vi "Dashboard Main.vi"() -> ()   [LabVIEW 2017]
uses:
  <vilib>/Utility/miscctls.llb/LVRowAndColumnTypeDef.ctl
  <vilib>/event_ctls.llb/eventvkey.ctl
  <vilib>/Rock Robotics/Network Tables/NT Read Numeric Array.vi
  <vilib>/Rock Robotics/Network Tables/NT Read Boolean.vi
  <vilib>/Rock Robotics/WPI/Dashboard/WPI_DashboardLogging Global.vi
  <vilib>/vision/NI_Vision_Development_Module.lvlib
panel:
  in  "Camera Settings Right":T1={"Frame Rate"=30, "Compression"=30, "Size"=1, "DB Camera Config"=FALSE} {"Frame Rate" scale=1.0..30.0; "Compression" scale=100.0..-1.0; "Size" items=["640x480", "320x240", "160x120"]}
  in  "Camera Name Right":string(combo)="No Camera Selection"
  out "Camera Info":cluster{"Mbps LED":bool, "Mbps":dbl, "fps":dbl} {"fps" format="%#.1g"; "Mbps" format="%#.1g"}
  in  "Camera Settings":T1={"Frame Rate"=30, "Compression"=30, "Size"=1, "DB Camera Config"=FALSE} {"Frame Rate" scale=1.0..30.0; "Compression" scale=100.0..-1.0; "Size" items=["640x480", "320x240", "160x120"]}
  in  "TCP":refnum<k5>
  in  "Rec Mode":enum32{"Stop", "Record", "Playback"}(radio)
  out "Robot IP":string
  out "Image Message":string="Timeout in Camera Communications"
  in  "Dashboard Tab":T2(tab)
  in  "Select Auto":string(combo)="Select Autonomous ..."
  out "NT Connection":bool
  out "MotorChart R":cluster{"Numeric":dbl, "Numeric":dbl}(graph)
  out "MotorChart L":cluster{"Numeric":dbl, "Numeric":dbl}(graph)
  out "MotorSliders R":cluster{"MotorSlide1":dbl, "MotorSlide2":dbl} {"MotorSlide2" scale=-1.0..1.0 scale format="%#_2e"; "MotorSlide1" scale=-1.0..1.0 scale format="%#_2e"}
  out "MotorSliders L":cluster{"MotorSlide1":dbl, "MotorSlide2":dbl} {"MotorSlide2" scale=-1.0..1.0 scale format="%#_2e"; "MotorSlide1" scale=-1.0..1.0 scale format="%#_2e"}
  out "Gyro":dbl(knob) scale=0.0..360.0
  out "JS1 Z":dbl(slide) scale=-1.0..1.0 scale format="%#_2e"
  out "JS1 Graph":cluster{"X":dbl, "Y":dbl}[](graph)
  out "JS1 Buttons":T3
  out "JS2 Z":dbl(slide) scale=-1.0..1.0 scale format="%#_2e"
  out "JS2 Graph":cluster{"X":dbl, "Y":dbl}[](graph)
  out "JS2 Buttons":T3
  out "Mode":T4(ring)=enum."Auto Disabled"
  out "Camera Image Right":T5(plugin-control)
  in  "DB/String 9":string
  in  "DB/String 8":string
  in  "DB/String 7":string
  in  "DB/String 6":string
  in  "DB/String 5":string
  in  "DB/String 4":string
  in  "DB/String 3":string
  in  "DB/String 2":string
  in  "DB/String 1":string
  in  "DB/String 0":string
  in  "DB/Slider 0":dbl(slide) scale=0.0..5.0
  in  "DB/Slider 1":dbl(slide) scale=0.0..5.0
  in  "DB/Slider 2":dbl(slide) scale=0.0..5.0
  in  "DB/Slider 3":dbl(slide) scale=0.0..5.0
  out "DB/LED 3":bool
  out "DB/LED 2":bool
  out "DB/LED 1":bool
  out "DB/LED 0":bool
  in  "DB/Button 3":bool
  in  "DB/Button 2":bool
  in  "DB/Button 1":bool
  in  "DB/Button 0":bool caption="New Name"
  in  "Drive X-Axis Correction":dbl=-0.2
  out "UseLeftEncoder":bool
  out "RDrive Encoder":dbl
  out "Flip Active":bool
  in  "BackCamera Rotate":sgl min=-360 max=360 step=1 format="%#_3g"
  in  "FrontCamera Rotate":sgl min=-360 max=360 step=1 format="%#_3g"
  out "Arm Sensor":bool
  out "Belly Sensor":bool
  out "Arm Encoder":dbl
  out "Arm Switch":bool
  out "LDrive Encoder":dbl
  in  "Test Slider":dbl(slide) scale=0.0..100.0 scale format="%#_3g"
  in  "On/Off":bool caption="Solenoid"
  in  "Test Name":u16(ring) items=["Select the test to run..."]
  in  "Test Tree":string(tree)
  in  "Motor":cluster{"Value":dbl, "Enable":bool} {"Value" scale=-1.0..1.0 scale format="%#_3g"}
  out "Progress":T6 {"Test Progress" scale=0.0..100.0}
  in  "Rev/Fwd":cluster{"Forward":bool, "Reverse":bool}
  in  "Test Ring":u16(ring) items=["Monochrome", "Color"]
  out "Cmd Status":string
  in  "Execute Command":bool
  in  "Command Params":string[][](table)
  in  "Command Selection":i32(listbox)
  in  "CheckList":i32(listbox)
  out "Tree":string(tree)
  out "Camera Image":T5(plugin-control)
  out "Background":bool
  in  "Camera Name":string(combo)="No Camera Selection"
  # "HW"
  # "HW"
  # "Joysticks"
  # "Drive Motors"
  # "Front"
  # "Right"
  # "Left"
  # "Back"
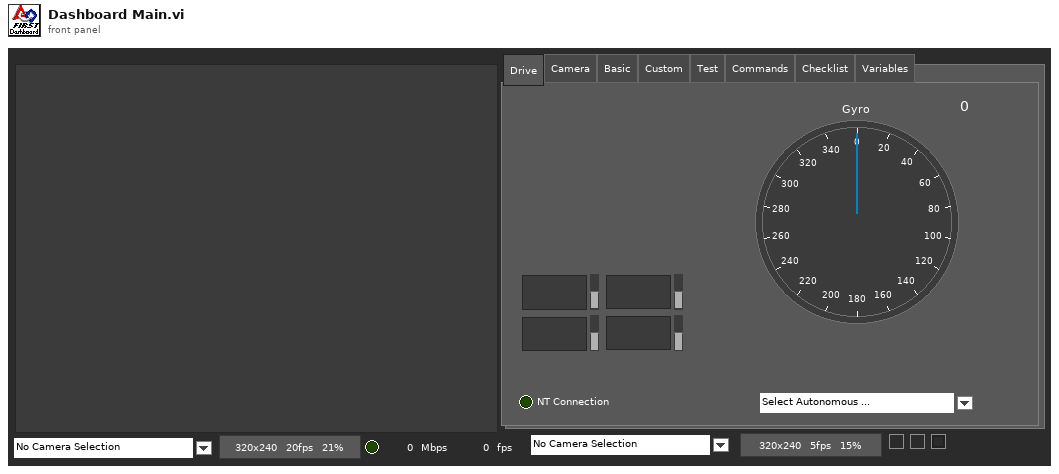
[diagram p1: front panel]
types:
  T1 = cluster{"Frame Rate":i32, "Compression":i32, "Size":u16, "DB Camera Config":bool}
  T2 = enum32{"Drive", "Camera", "Basic", "Custom", "Test", "Commands", "Checklist", "Variables"}
  T3 = cluster{bool, bool, bool, bool, bool, bool, bool, bool, bool, bool, bool, bool}
  T4 = enum8{"Tele-Op Disabled", "Tele-Op Enabled", "Auto Disabled", "Auto Enabled", "Test Disabled", "Test Enabled", "Disconnected", "No Code", "E-Stop"}
  T5 = typedef "IMAQ Image.ctl" = refnum<image>
  T6 = cluster{"Test Progress":u8, "Test Progress Text":string}
  T7 = cluster{"Save Path":path, "Interval (s)":dbl, "Keep":i32}
  T8 = typedef "Image Type" = u32
  T9 = cluster{"IDs":cluster{"RPC field ID":u16, "Unique ID":u16}, "String":string}
  T10 = cluster{string, string, "Saved DB Images Info":cluster{"Save Path":path, "Interval (s)":dbl, "Keep":i32}}
  T11 = cluster{"Camera Image":refnum<vi>, "Dashboard Tab":refnum<vi>, "Background":refnum<vi>, "Rec Mode":refnum<vi>, "Test Slider":refnum<vi>, "On/Off ":refnum<vi>, "Test Ring":refnum<vi>, "Rev/Fwd":refnum<vi>, "Test Name":refnum<vi>, "Motor":refnum<vi>, "Progress":refnum<vi>, "CheckList":refnum<vi>, "Tree":refnum<vi>, "Test Tree":refnum<vi>, "Command Params":refnum<vi>, "Command Selection":refnum<vi>, "Execute Command":refnum<vi>, "Cmd Status":refnum<vi>, "Camera Settings":refnum<vi>, "Camera Name":refnum<vi>, "Camera Info":refnum<vi>, "Camera Settings Right":refnum<vi>, "Camera Name Right":refnum<vi>, "Camera Image Right":refnum<vi>}
  T12 = cluster{"Error Strings":string, "Disable Counts":cluster{u16, u16}, "Rail Faults":cluster{u16, u16, u16}, "Robot IP":string, "DB Mode":u8, "Event Info":cluster{"Name":string, "Type":u8, "Number":u16, "Replay":u8}}
  T13 = cluster{"Storage":cluster{"Disk Free":u64, "RAM Block":u32, "RAM free":u32}, "CPU Utilization":cluster{"CPU % ISR":sgl, "CPU % Time Crit":sgl, "CPU % Timed Str":sgl, "CPU % High":sgl, "CPU % Above":sgl, "CPU % Normal":sgl, "CPU % Low":sgl}, "CAN":cluster{"% Bus Utilization":sgl, "Bus Off Cnt":u32, "TX_FIFO Full Cnt":u32, "Receive Error Cnt":u8, "Transmit Error Cnt":u8}, "HID":cluster{"HID Outputs":u32, "Rumble Low":u16, "Rumble High":u16}[]}
  T14 = cluster{"Status bits":cluster{"Test Mode":bool, "Autonomous":bool, "Enabled":bool, "Code Start":bool, "Brownout":bool, "Reserved 2":bool, "Reserved 3":bool, "E-Stop":bool}, "Code Trace":cluster{"Disabled":bool, "TeleOp":bool, "Auto":bool, "Test":bool}, "Controller Type":enum16{"unknown", "cRIO", "roboRio"}, "Code?":enum16{"unknown", "noCode", "code"}, "Battery V":dbl}
  T15 = cluster{"Control Bits":cluster{"TestMode":bool, "Autonomous":bool, "Enabled":bool, "FMS Present":bool, bool, bool, bool, "E-Stop":bool}, "Team Station ":u8, "Countdown":sgl, "Joystick Values":cluster{"Axes":dbl[], "Buttons":bool[], "POVs":i16[]}[]}
  T16 = cluster{"Axes":dbl[], "Buttons":bool[], "POVs":i16[]}[]
  T17 = cluster{"Axes":dbl[], "Buttons":bool[], "POVs":i16[]}
  T18 = cluster{"Buttons[0]":bool, "Buttons[1]":bool, "Buttons[2]":bool, "Buttons[3]":bool, "Buttons[4]":bool, "Buttons[5]":bool, "Buttons[6]":bool, "Buttons[7]":bool, "Buttons[8]":bool, "Buttons[9]":bool, "Buttons[10]":bool, "Buttons[11]":bool}
  T19 = cluster{"Camera Name Right":string, string, "Saved DB Images Info":cluster{"Save Path":path, "Interval (s)":dbl, "Keep":i32}}
  T20 = cluster{"Operation":enum16{"Update", "Clear"}, "Color Box":u32}[]
  T21 = typedef "eventvkey.ctl" = enum16{"ASCII", "Enter", "Return", "Shift", "Ctrl", "Alt", "Cmd", "Opt", "Caps", "NumLock", "Clear", "Break", "Up", "Down", "Left", "Right", "Insert", "Delete", "Home", "End", "PageUp", "PageDown", "Escape", "Help", "Pause", "ScrollLock", "F1", "F2", "F3", "F4", "F5", "F6", "F7", "F8", "F9", "F10", "F11", "F12", "F13", "F14", "F15", "F16", "F17", "F18", "F19", "F20", "F21", "F22", "F23", "F24", "Play", "VolumeUp", "VolumeDown", "Mute", "Two Byte Char"}
  T22 = cluster{"Image Size":bool, "Image Type":bool, "Pixel Value":bool, "ROI Information":bool, "Zoom Factor":bool}
  T23 = cluster{"Operation":enum16{"Update", "Clear"}, "Color Box":u32}
  T24 = typedef "LVRowAndColumnTypeDef.ctl" = cluster{"Row":i32, "Column":i32}
  T25 = cluster{"Shift":bool, "Ctrl":bool, "Alt":bool, "Cmd":bool, "Opt":bool}
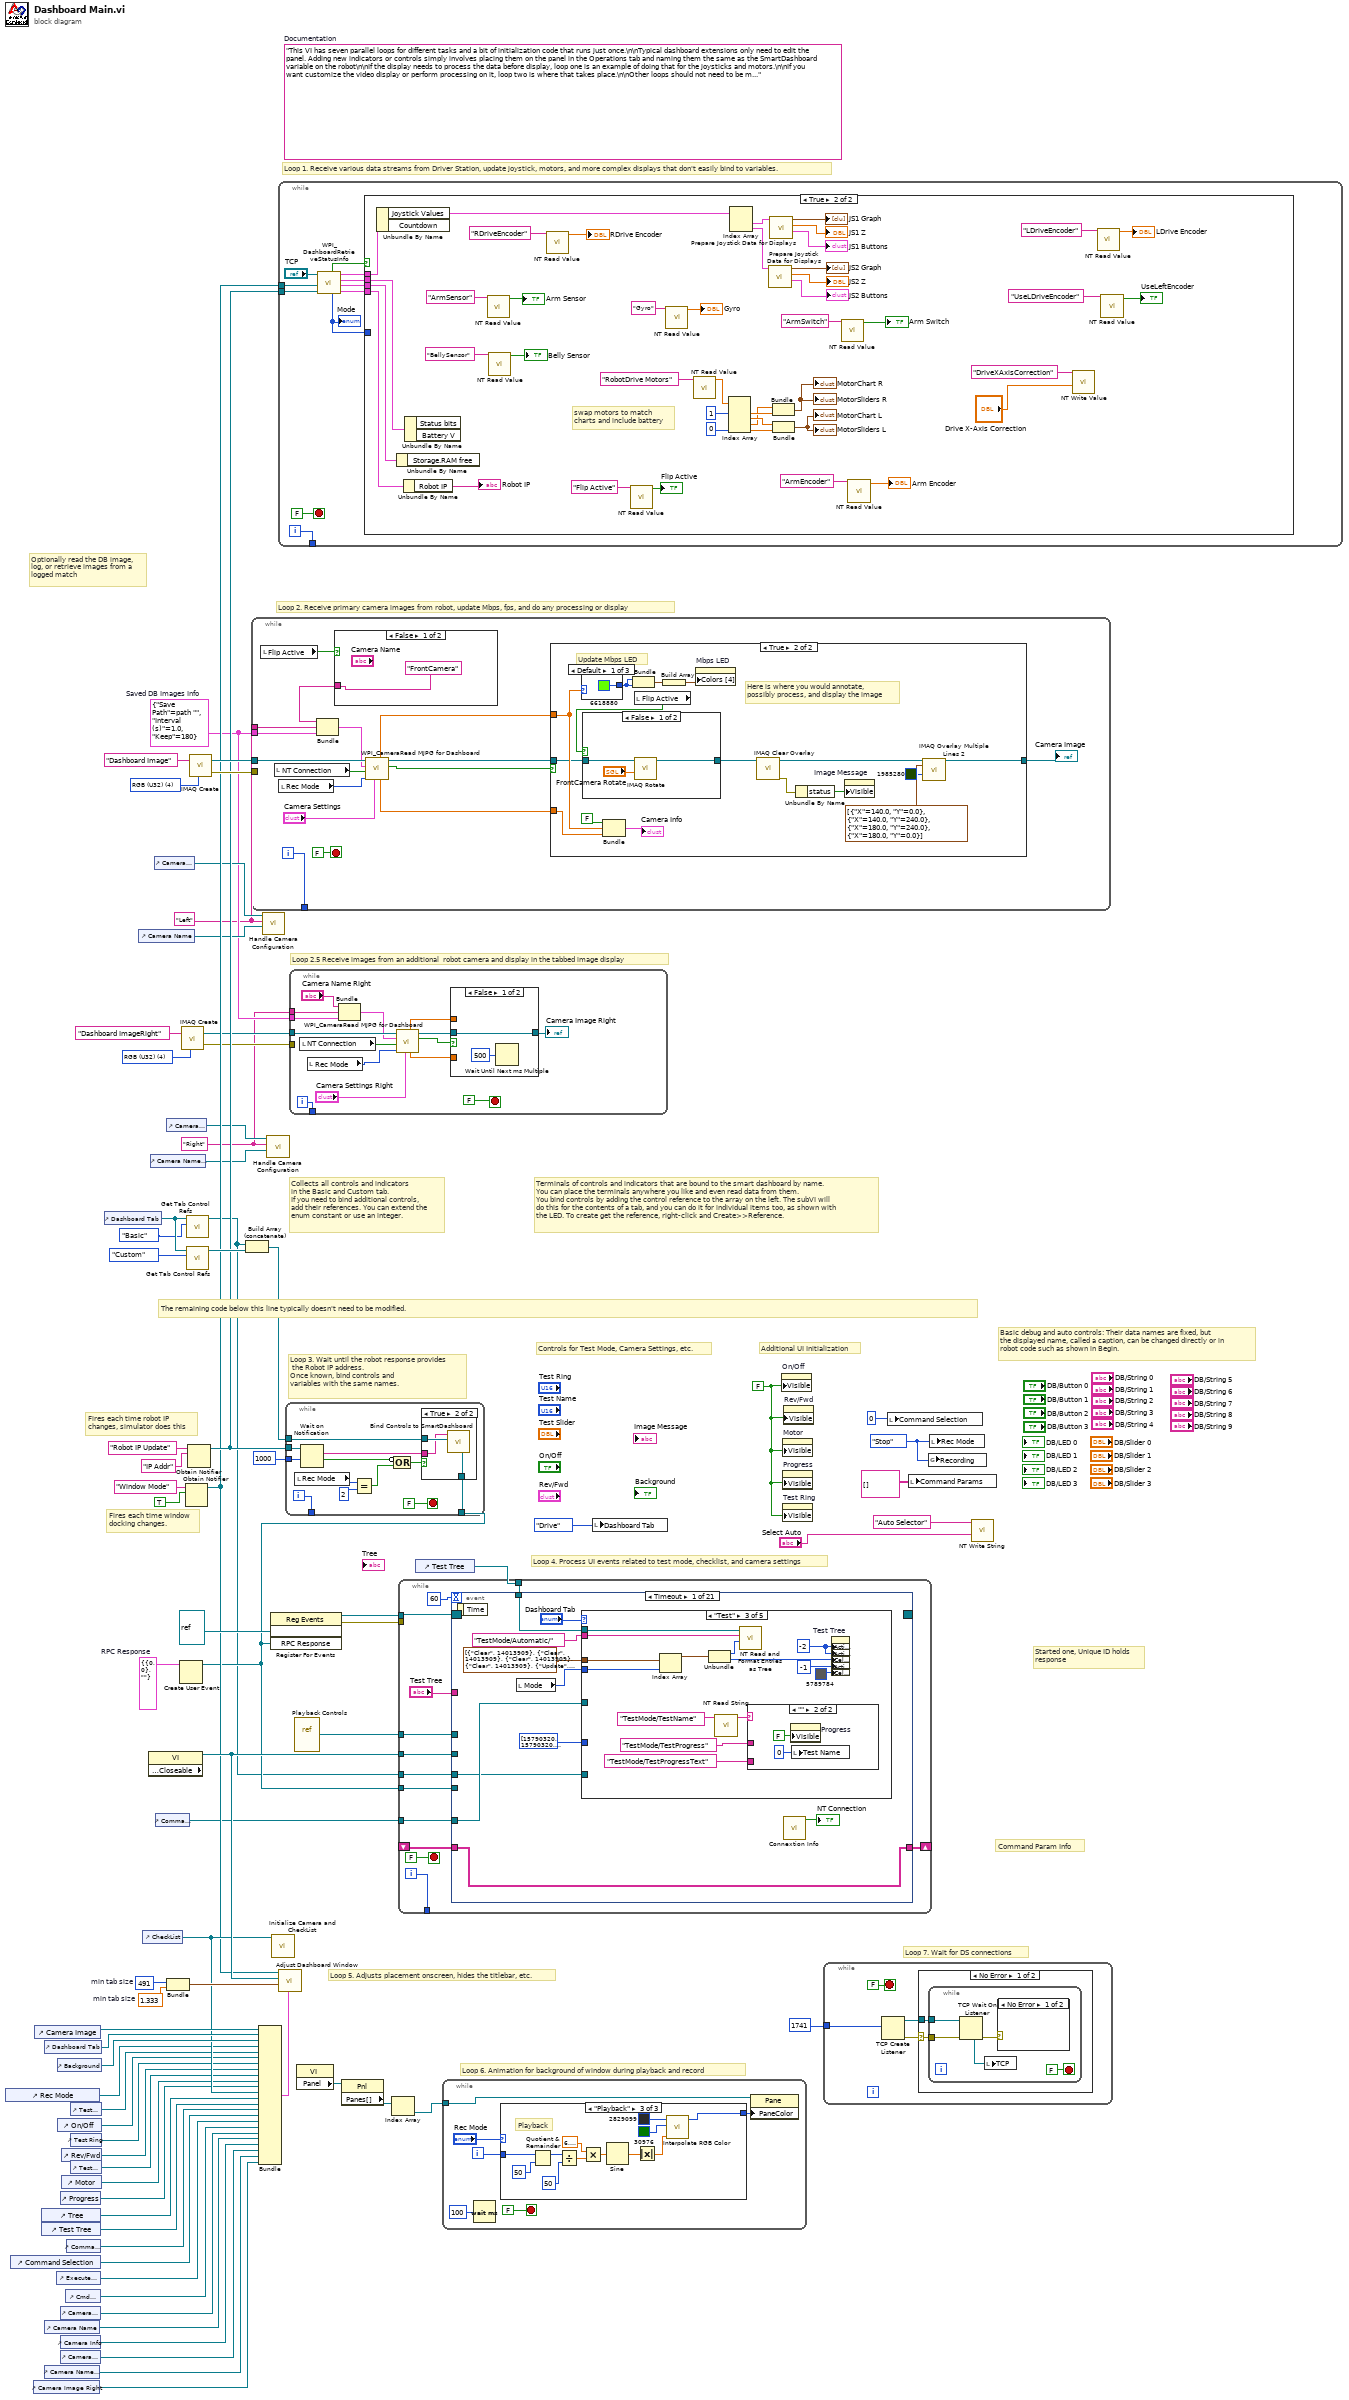
[diagram p0: block diagram]
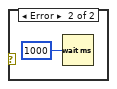
[diagram p3: hidden frame]
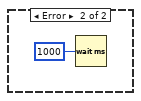
[diagram p4: hidden frame]
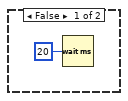
[diagram p5: hidden frame]
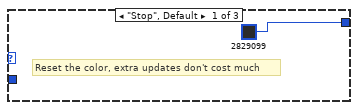
[diagram p6: hidden frame]
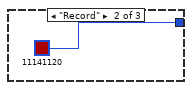
[diagram p7: hidden frame]
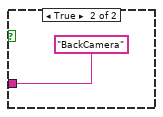
[diagram p9: hidden frame]
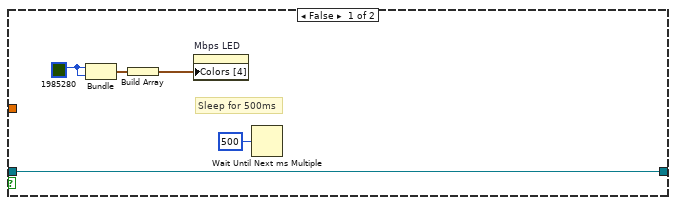
[diagram p10: hidden frame]
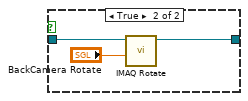
[diagram p11: hidden frame]
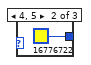
[diagram p12: hidden frame]
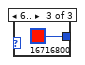
[diagram p13: hidden frame]
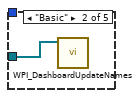
[diagram p15: hidden frame]
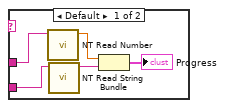
[diagram p16: hidden frame]
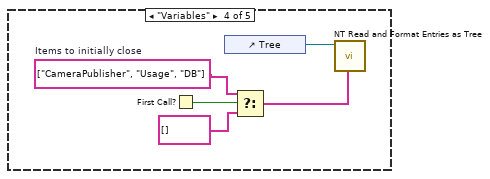
[diagram p17: hidden frame]
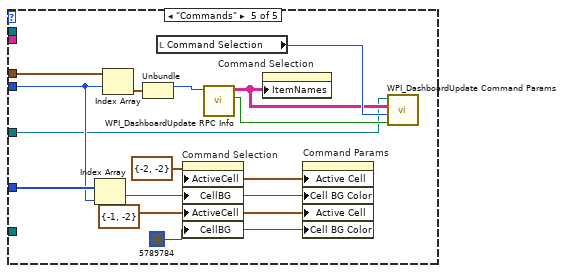
[diagram p18: hidden frame]
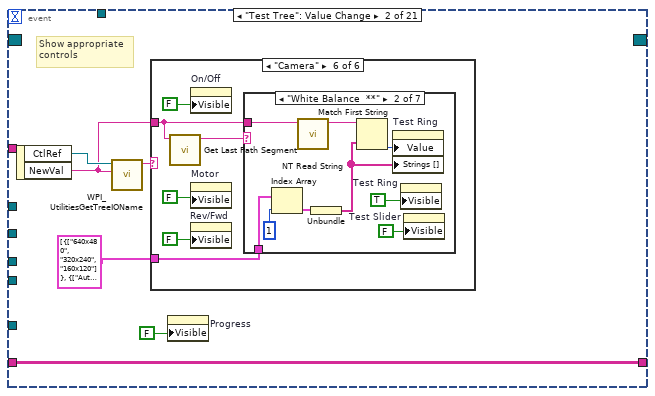
[diagram p19: hidden frame]
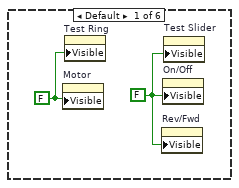
[diagram p20: hidden frame]
diagram:
  w4 = T7 {"Save Path"=path "", "Interval (s)"=1.0, "Keep"=180}  # Saved DB Images Info
  w3 = "Right"
  w2 = "Left"
  w14 = T8 4 items=["Grayscale (U8)", "Grayscale (I16)", "Grayscale (SGL)", "Complex (CSG)", "RGB (U32)", "HSL (U32)", "RGB (U64)"] ("Image Type")
  w29 = T9 {"IDs"={"RPC field ID"=0, "Unique ID"=0}, "String"=""}  # RPC Response
  w52 = 491  # min tab size
  w51 = 1.333  # min tab size
  w59 = enum32{"Stop", "Record", "Playback"}."Stop" ("Rec Mode")
  w36 = FALSE ("Visible")
  (unwired) "This VI has seven parallel loops for different tasks and a bit of initialization code that runs just once.\n\nTypical dashboard extensions only need to edit the panel. Adding new indicators or controls simply involves placing them on the panel in the Operations tab and naming them the same as the SmartDashboard variable on the robot\n\nIf the display needs to process the data before display, loop one is an example of doing that for the joysticks and motors.\n\nIf you want customize the video display or perform processing on it, loop two is where that takes place.\n\nOther loops should not need to be modified. They are pretty standard, and document the task they perform."  # Documentation
  w76 = T8 4 items=["Grayscale (U8)", "Grayscale (I16)", "Grayscale (SGL)", "Complex (CSG)", "RGB (U32)", "HSL (U32)", "RGB (U64)"] ("Image Type")
  # "Optionally read the DB image,\nlog, or retrieve images from a\nlogged match"
  # "Loop 2.5 Receive images from an additional  robot camera and display in the tabbed image display"
  # "Command Param Info"
  # "Started one, Unique ID holds\nresponse"
  # "Loop 7. Wait for DS connections"
  # "Basic debug and auto controls: Their data names are fixed, but\nthe displayed name, called a caption, can be changed directly or in\nrobot code such as shown in Begin."
  # "Controls for Test Mode, Camera Settings, etc."
  # "Additional UI Initialization"
  # "Loop 6. Animation for background of window during playback and record"
  # "Fires each time robot IP\nchanges, simulator does this"
  # "Fires each time window\ndocking changes."
  # "Collects all controls and indicators\nin the Basic and Custom tab.\nIf you need to bind additional controls,\nadd their references. You can extend the\nenum constant or use an integer."
  # "The remaining code below this line typically doesn't need to be modified."
  # "Loop 4. Process UI events related to test mode, checklist, and camera settings"
  # "Terminals of controls and indicators that are bound to the smart dashboard by name.\nYou can place the terminals anywhere you like and even read data from them.\nYou bind controls by adding the control reference to the array on the left. The subVI will\ndo this for the contents of a tab, and you can do it for individual items too, as shown with\nthe LED. To create get the reference, right-click and Create>>Reference."
  # "Loop 3. Wait until the robot response provides\n the Robot IP address.\nOnce known, bind controls and\nvariables with the same names."
  # "Loop 5. Adjusts placement onscreen, hides the titlebar, etc."
  # "Loop 1. Receive various data streams from Driver Station, update joystick, motors, and more complex displays that don't easily bind to variables."
  # "Loop 2. Receive primary camera images from robot, update Mbps, fps, and do any processing or display"
  n1 = control-ref of="Rec Mode"() -> (w42:refnum<vi>)
  n2 = control-ref of="Command Selection"() -> (w28:refnum<vi>)
  n3 = control-ref of="Camera Image Right"() -> (w7:refnum<vi>)
  n4 = control-ref of="Camera Image"() -> (w54:refnum<vi>)
  n5 = control-ref of="Tree"() -> (w46:refnum<vi>)
  n6 = control-ref of="Test Tree"() -> (w45:refnum<vi>)
  n7 = control-ref of="Dashboard Tab"() -> (w53:refnum<vi>)
  n8 = control-ref of="Camera Name"() -> (w19:refnum<vi>)
  n9 = control-ref of="Camera Name Right"() -> (w8:refnum<vi>)
  n10 = control-ref of="Execute Command"() -> (w30:refnum<vi>)
  n11 = control-ref of="Background"() -> (w49:refnum<vi>)
  n12 = control-ref of="On/Off"() -> (w40:refnum<vi>)
  n13 = control-ref of="Progress"() -> (w37:refnum<vi>)
  n14 = control-ref of="Camera Settings"() -> (w20:refnum<vi>)
  n15 = control-ref of="Camera Info"() -> (w18:refnum<vi>)
  n16 = control-ref of="Camera Settings Right"() -> (w9:refnum<vi>)
  n17 = control-ref of="Rev/Fwd"() -> (w38:refnum<vi>)
  n18 = control-ref of="Motor"() -> (w43:refnum<vi>)
  n19 = control-ref of="Cmd Status"() -> (w24:refnum<vi>)
  n20 = control-ref of="Command Params"() -> (w31:refnum<vi>)
  n21 = control-ref of="Test Slider"() -> (w41:refnum<vi>)
  n22 = control-ref of="Test Ring"() -> (w39:refnum<vi>)
  n23 = control-ref of="Test Name"() -> (w44:refnum<vi>)
  n24 = control-ref of="Dashboard Tab"() -> (w57:refnum<vi>)
  n25 = control-ref of="Camera Name"() -> (w21:refnum<vi>)
  n26 = control-ref of="CheckList"() -> (w47:refnum<vi>)
  n27 = property class="VI" props=["Front Panel.Closeable"]() -> (reference out=w58:refnum<vi>)  [unwired: 2 in, 2 out]
  n28 = control-ref of="Camera Name Right"() -> (w10:refnum<vi>)
  n29 = control-ref of="Camera Settings"() -> (w22:refnum<vi>)
  n30 = control-ref of="Command Params"() -> (w23:refnum<vi>)
  n31 = control-ref of="Camera Settings Right"() -> (w11:refnum<vi>)
  n32 = Bundle("min tab size"=w52, "min tab size"=w51) -> (w50:cluster{"min tab size":i32, "min tab size":dbl})  [unwired: 1 in]
  n33 = Create User Event(user event datatype=w29) -> (user event=w25:refnum<user-event>)  [unwired: 1 in, 1 out]
  n34 = call "IMAQ Create"("Image Name"="Dashboard ImageRight", "Image Type"=w14) -> ("New Image"=w13:T5, "error out"=w12:errorcluster)  [unwired: 2 in, 1 out]
  n35 = Obtain Notifier(name (unnamed)="Window Mode", notification data type=TRUE) -> (notifier out=w34:refnum<notifier>)  [unwired: 2 in, 2 out]
  n36 = call <vilib>:"Get Tab Control Refs.vi"("Page Index"=T2."Basic" ("Dashboard Tab"), "TabControl in"=w57) -> ("ControlsOnPage"=w17:refnum<vi>[])  [unwired: 9 in]
  n37 = call <vilib>:"Get Tab Control Refs.vi"("Page Index"=T2."Custom" ("Dashboard Tab"), "TabControl in"=w57) -> ("ControlsOnPage"=w56:refnum<vi>[])  [unwired: 9 in]
  n38 = Obtain Notifier(name (unnamed)="Robot IP Update", notification data type="IP Addr" ("name (unnamed)")) -> (notifier out=w35:refnum<notifier>)  [unwired: 2 in, 2 out]
  n39 = call "IMAQ Create"("Image Name"="Dashboard Image", "Image Type"=w76) -> ("New Image"=w74:T5, "error out"=w73:errorcluster)  [unwired: 2 in, 1 out]
  n40 = Build Array (concatenate)(w17, w56) -> (w55:refnum<vi>[])
  n41 = while {
    tunnel: w74 -> [w90]
    tunnel: w73 -> [_]
    tunnel: [w91] -> _
    tunnel: w4 -> [w81]
    tunnel: w2 -> [w80]
    i -> [w91]
    stop <- FALSE stop-if-true
    n42 = local read "Flip Active"() -> (w77:bool)
    n43 = local read "NT Connection"() -> (w82:bool)
    n44 = local read "Rec Mode"() -> (w86:enum32{"Stop", "Record", "Playback"})
    n45 = case shown="False" w77 {
      tunnel: ["FrontCamera" "BackCamera"] -> w79
      frame False {
      }
      frame True {
      }
    }
    n46 = Bundle(w79, w80, "Saved DB Images Info"=w81) -> (w78:T10)  [unwired: 1 in]
    n47 = call <vilib>:"WPI_CameraRead MJPG for Dashboard.vi"("Camera Settings"="Camera Settings", "Rec Mode"=w86, "NT Connection"=w82, "Capture Info"=w78, "Refnum in"=w90) -> ("Active"=w88:bool, "Refnum out"=w89:T5, "FPS"=w87:dbl, "Bandwidth (Mbps)"=w85:dbl)  [unwired: 3 in]
    n48 = case shown="True" w88 {
      tunnel: w89 -> [w95 w102]
      tunnel: w85 -> [_ w109]
      tunnel: w87 -> [_ w110]
      tunnel: [w95 w105] -> w83
      frame False {
        w97 = u32 1985280 ("Color Box")
        # "Sleep for 500ms"
        n49 = Bundle("Color Box"=w97, "Color Box"=w97) -> (w98:cluster{"Color Box":u32, "Color Box":u32})  [unwired: 1 out]
        n50 = Build Array(w98) -> (w96:cluster{"Color Box":u32, "Color Box":u32}[])
        n51 = property on="Mbps LED" class="Bool (strict)"("Colors [4]"=w96) -> ()  [unwired: 2 in, 2 out]
        n52 = Wait Until Next ms Multiple(millisecond multiple=u32 500) -> ()  [unwired: 1 out]
      }
      frame True {
        # "Here is where you would annotate,\npossibly process, and display the image"
        # "Update Mbps LED"
        n53 = case shown="Default" w109 {
          tunnel: [u32 6618880 ("Color Box") u32 16776722 ("Color Box") u32 16716800 ("Color Box")] -> w112
          frame Default {
          }
          frame 4, 5 {
          }
          frame 6.. {
          }
        }
        n54 = Bundle(FALSE, "Bandwidth (Mbps)"=w109, "FPS"=w110) -> (→"Camera Info":cluster{bool, "Bandwidth (Mbps)":dbl, "FPS":dbl})  [unwired: 1 in]
        n55 = Bundle("Color Box"=w112, "Color Box"=w112) -> (w113:cluster{"Color Box":u32, "Color Box":u32})  [unwired: 1 out]
        n56 = local read "Flip Active"() -> (w100:bool)
        n57 = case shown="False" w100 {
          tunnel: w102 -> [w118 w121]
          tunnel: [w117 w120] -> w101
          frame False {
            n58 = call "IMAQ Rotate"("Angle (degrees)"="FrontCamera Rotate", "Image Src"=w118) -> ("Image Dst Out"=w117:T5)  [unwired: 8 in, 1 out]
          }
          frame True {
            n59 = call "IMAQ Rotate"("Angle (degrees)"="BackCamera Rotate", "Image Src"=w121) -> ("Image Dst Out"=w120:T5)  [unwired: 8 in, 1 out]
          }
        }
        n60 = Build Array(w113) -> (w111:cluster{"Color Box":u32, "Color Box":u32}[])
        n61 = property on="Mbps LED" class="Bool (strict)"("Colors [4]"=w111) -> ()  [unwired: 2 in, 2 out]
        n62 = call "IMAQ Clear Overlay"("Image"=w101) -> ("error out"=w114:errorcluster, "Image Out"=w106:T5)  [unwired: 2 in, 7 out]
        n63 = Unbundle By Name(w114) -> ("status"=w115:bool)
        n64 = property on="Image Message" class="Str"("Visible"=w115) -> ()  [unwired: 2 in, 2 out]
        n65 = call "IMAQ Overlay Multiple Lines 2"("Image"=w106, "Line End Points"=cluster{"X":dbl, "Y":dbl}[] [{"X"=140.0, "Y"=0.0}, {"X"=140.0, "Y"=240.0}, {"X"=180.0, "Y"=240.0}, {"X"=180.0, "Y"=0.0}], "Color"=u32 1985280) -> ("Image Out"=w105:T5)  [unwired: 11 in, 1 out]
      }
    }
    "Camera Image" <- w83
  }
  n66 = Bundle("Camera Image"=w54, "Dashboard Tab"=w53, "Background"=w49, "Rec Mode"=w42, "Test Slider"=w41, "On/Off"=w40, "Test Ring"=w39, "Rev/Fwd"=w38, "Test Name"=w44, "Motor"=w43, "Progress"=w37, "CheckList"=w47, "Tree"=w46, "Test Tree"=w45, "Command Params"=w31, "Command Selection"=w28, "Execute Command"=w30, "Cmd Status"=w24, "Camera Settings"=w20, "Camera Name"=w19, "Camera Info"=w18, "Camera Settings Right"=w9, "Camera Name Right"=w8, "Camera Image Right"=w7) -> (w48:T11)  [unwired: 1 in]
  n67 = call "Handle Camera Configuration.vi"("CameraNameRef"=w21, "Display Name"=w2, "ClusterRef"=w22) -> ()  [unwired: 9 in]
  n68 = call "Handle Camera Configuration.vi"("CameraNameRef"=w10, "Display Name"=w3, "ClusterRef"=w11) -> ()  [unwired: 9 in]
  n69 = register-events(refnum<vi> refnum, w25) -> (reference out=w63:refnum<event-registration>, error out=w62:errorcluster)  [unwired: 2 in]
  n70 = call "Initialize Camera and CheckList.vi"("ListBox in"=w47) -> ()  [unwired: 11 in]
  n71 = while {
    tunnel: [w134] -> _
    tunnel: w35 -> [w128]
    tunnel: w34 -> [w125]
    i -> [w134]
    stop <- FALSE stop-if-true
    n72 = call <vilib>:"WPI_DashboardRetrieveStatusInfo.vi"("Binding Refnum"=w128, "Window Mode Notifier"=w125, "TCP Cnx"="TCP") -> ("Power and Errors"=w129:T12, "Robot Metrics"=w132:T13, "Status Info"=w133:T14, "Control Info"=w130:T15, "Robot Mode"=w127:T4, "Process?"=w131:bool)  [unwired: 3 in]
    "Mode" <- w127
    n73 = case shown="True" w131 {
      tunnel: w133 -> [_ w180]
      tunnel: w132 -> [_ w179]
      tunnel: w130 -> [_ w178]
      tunnel: w129 -> [_ w177]
      tunnel: w127 -> [_ _]
      frame False {
        n74 = Wait (ms)(milliseconds to wait=u32 20) -> ()  [unwired: 1 out]
      }
      frame True {
        # "swap motors to match\ncharts and include battery"
        n75 = Unbundle By Name(w178) -> ("Joystick Values"=w168:T16)  [unwired: 1 out]
        n76 = Unbundle By Name(w179) -> ()  [unwired: 1 out]
        n77 = Unbundle By Name(w177) -> ("Robot IP"=→"Robot IP":string)
        n78 = Unbundle By Name(w180) -> ()  [unwired: 2 out]
        n79 = call-poly <vilib>:"NT Read Value.vi"("Name"="ArmSensor") -> ("Boolean"=→"Arm Sensor":bool)  [unwired: 9 in, 1 out]
        n80 = call-poly <vilib>:"NT Read Value.vi"("Name"="BellySensor") -> ("Boolean"=→"Belly Sensor":bool)  [unwired: 9 in, 1 out]
        n81 = call-poly <vilib>:"NT Read Value.vi"("Name"="RDriveEncoder") -> ("Numeric"=→"RDrive Encoder":dbl)  [unwired: 9 in, 1 out]
        n82 = call-poly <vilib>:"NT Read Value.vi"("Name"="Flip Active") -> ("Boolean"=→"Flip Active":bool)  [unwired: 9 in, 1 out]
        n83 = call-poly <vilib>:"NT Read Value.vi"("Name"="Gyro") -> ("Numeric"=→"Gyro":dbl)  [unwired: 9 in, 1 out]
        n84 = call-poly <vilib>:"NT Read Value.vi"("Name"="RobotDrive Motors") -> ("Numeric Array"=w158:dbl[])  [unwired: 9 in, 1 out]
        n85 = Index Array(array=w158, index #1=1, index #4=0) -> (element #1=w172:dbl, element #2=w173:dbl, element #3=w171:dbl, element #4=w176:dbl)  [unwired: 2 in]
        n86 = Index Array(array=w168) -> (element #1=w167:T17, element #2=w163:T17)  [unwired: 2 in]
        n87 = call "Prepare Joystick Data for Displays.vi"("Joystick Values"=w163) -> ("Buttons"=→"JS2 Buttons":T18, "Z Axis"=→"JS2 Z":dbl, "Cartesian Data"=→"JS2 Graph":cluster{"X axis":dbl, "X axis":dbl}[])  [unwired: 8 in]
        n88 = call "Prepare Joystick Data for Displays.vi"("Joystick Values"=w167) -> ("Buttons"=→"JS1 Buttons":T18, "Z Axis"=→"JS1 Z":dbl, "Cartesian Data"=→"JS1 Graph":cluster{"X axis":dbl, "X axis":dbl}[])  [unwired: 8 in]
        n89 = Bundle("Numeric"=w171, "Numeric"=w172) -> (→"MotorChart R" →"MotorSliders R":cluster{"Numeric":dbl, "Numeric":dbl})  [unwired: 1 in]
        n90 = Bundle("Numeric"=w173, "Numeric"=w176) -> (→"MotorChart L" →"MotorSliders L":cluster{"Numeric":dbl, "Numeric":dbl})  [unwired: 1 in]
        n91 = call-poly <vilib>:"NT Read Value.vi"("Name"="ArmSwitch") -> ("Boolean"=→"Arm Switch":bool)  [unwired: 9 in, 1 out]
        n92 = call-poly <vilib>:"NT Read Value.vi"("Name"="ArmEncoder") -> ("Numeric"=→"Arm Encoder":dbl)  [unwired: 9 in, 1 out]
        n93 = call-poly <vilib>:"NT Write Value.vi"("Numeric"="Drive X-Axis Correction", "Name"="DriveXAxisCorrection") -> ()  [unwired: 9 in, 1 out]
        n94 = call-poly <vilib>:"NT Read Value.vi"("Name"="LDriveEncoder") -> ("Numeric"=→"LDrive Encoder":dbl)  [unwired: 9 in, 1 out]
        n95 = call-poly <vilib>:"NT Read Value.vi"("Name"="UseLDriveEncoder") -> ("Boolean"=→"UseLeftEncoder":bool)  [unwired: 9 in, 1 out]
      }
    }
  }
  n96 = call "Adjust Dashboard Window.vi"("Sizing Refnums"=w48, "Size Constraints"=w50, "VI"=w58, "WIn Mode"=w34) -> ()  [unwired: 8 in]
  n97 = while {
    tunnel: w55 -> [w192]
    tunnel: w35 -> [w190]
    tunnel: [w188] -> _
    tunnel: u32 1000 ("milliseconds to wait") -> [w187]
    tunnel: w25 -> [w181]
    i -> [w188]
    stop <- FALSE stop-if-true
    n98 = local read "Rec Mode"() -> (w183:enum32{"Stop", "Record", "Playback"})
    n99 = Wait on Notification(notifier=w190, timeout in ms (-1)=w187) -> (notification=w189:string, timed out?=w185:bool)  [unwired: 2 in, 2 out]
    n100 = Equal?(x=w183, y=u16 2 ("Rec Mode")) -> (x = y?=w184:bool)
    n101 = Compound Arithmetic op=OR(invert w185, w184) -> (w186:bool)
    n102 = case shown="True" w186 {
      tunnel: w192 -> [_ w195]
      tunnel: w189 -> [_ w194]
      tunnel: w181 -> [_ w193]
      frame False {
      }
      frame True {
        n103 = call <vilib>:"Bind Controls to SmartDashboard.vi"("RPC ref"=w193, "Bound Control Refs"=w195, "Server IP Address"=w194) -> ()  [unwired: 9 in]
      }
    }
  }
  n104 = while {
    tunnel: w13 -> [w210]
    tunnel: w12 -> [_]
    tunnel: [w205] -> _
    tunnel: w4 -> [w199]
    tunnel: w3 -> [w196]
    i -> [w205]
    stop <- FALSE stop-if-true
    n105 = local read "NT Connection"() -> (w200:bool)
    n106 = local read "Rec Mode"() -> (w209:enum32{"Stop", "Record", "Playback"})
    n107 = Bundle("Camera Name Right"="Camera Name Right", w196, "Saved DB Images Info"=w199) -> (w198:T19)  [unwired: 1 in]
    n108 = call <vilib>:"WPI_CameraRead MJPG for Dashboard.vi"("Camera Settings"="Camera Settings Right", "Rec Mode"=w209, "NT Connection"=w200, "Capture Info"=w198, "Refnum in"=w210) -> ("Active"=w204:bool, "Refnum out"=w207:T5, "FPS"=w202:dbl, "Bandwidth (Mbps)"=w203:dbl)  [unwired: 3 in]
    n109 = case shown="False" w204 {
      tunnel: w207 -> [w211 w213]
      tunnel: w203 -> [_ _]
      tunnel: w202 -> [_ _]
      tunnel: [w211 w213] -> w201
      frame False {
        n110 = Wait Until Next ms Multiple(millisecond multiple=u32 500) -> ()  [unwired: 1 out]
      }
      frame True {
      }
    }
    "Camera Image Right" <- w201
  }
  n111 = vi-ref "Playback Controls.vi"() -> (w64:refnum<vi>)
  n112 = property class="VI"() -> ("Panel"=w66:refnum<vi>)  [unwired: 2 in, 2 out]
  n113 = property class="Pnl"(reference=w66) -> ("Panes[]"=w67:refnum<vi>[])  [unwired: 1 in, 2 out]
  n114 = Index Array(array=w67) -> (element=w65:refnum<vi>)  [unwired: 1 in]
  n115 = control-ref of="Test Tree"() -> (w68:refnum<vi>)
  n116 = while {
    tunnel: [w223] -> _
    tunnel: w68 -> [w222]
    tunnel: w64 -> [w221]
    tunnel: w63 -> [w220]
    tunnel: w62 -> [_]
    tunnel: w58 -> [w219]
    tunnel: w25 -> [w218]
    tunnel: w23 -> [w217]
    shift-right: [w216] -> _
    shift-left: _ -> [w215]
    tunnel: w17 -> [w214]
    i -> [w223]
    stop <- FALSE stop-if-true
    n117 = event shown="[0] Timeout" {
      selector: w220 -> [_ _ _ _ _ _ _ _ _ _ _ _ _ _ _ _ _ _ _ _ _]
      dyn-events: [_ _ _ _ _ _ _ _ _ _ _ _ _ _ _ _ w483 _ _ _ _] -> _
      timeout: u32 60 ("milliseconds to wait") -> [_ _ _ _ _ _ _ _ _ _ _ _ _ _ _ _ _ _ _ _ _]
      tunnel: w222 -> [w235 _ _ _ _ _ _ _ _ _ _ _ _ _ _ _ _ _ _ _ _]
      tunnel: "Test Tree" -> [_ _ _ _ _ _ _ _ _ _ _ w450 w458 w460 w464 w472 _ _ _ _ _]
      tunnel: w221 -> [_ _ _ _ _ _ _ _ _ _ _ _ _ _ _ _ w485 _ w503 _ _]
      tunnel: w219 -> [_ _ _ _ _ _ _ _ _ _ _ _ _ _ _ _ w481 _ _ _ _]
      tunnel: w218 -> [_ _ _ _ _ _ _ _ _ _ _ _ _ _ _ _ w479 _ _ _ _]
      tunnel: w217 -> [w230 _ _ _ _ _ w401 _ _ _ _ _ _ _ _ _ _ _ _ _ _]
      tunnel: [w229 w278 w380 w385 w394 w398 w399 w408 w418 w425 w437 w449 w456 w459 w463 w471 w478 w498 w500 w504 w517] -> w216
      tunnel: w215 -> [w229 w278 w380 w385 w394 w398 w399 _ _ w425 w437 w449 w456 w459 w463 w471 w478 w498 w500 w504 w517]
      tunnel: w214 -> [w227 _ _ _ _ _ _ _ _ _ _ _ _ _ _ _ _ _ _ _ _]
      event Timeout {
        n118 = event-data() -> ()  [unwired: 1 in, 1 out]
        n119 = local read "Mode"() -> (w232:T4)
        n120 = case shown="\"Test\"" "Dashboard Tab" {
          tunnel: w235 -> [_ _ w251 _ _]
          tunnel: "TestMode/Automatic/" ("Name Pattern") -> [_ _ w250 _ _]
          tunnel: T20 [{"Operation"=enum."Clear", "Color Box"=14013909}, {"Operation"=enum."Clear", "Color Box"=14013909}, {"Operation"=enum."Clear", "Color Box"=14013909}, {"Operation"=enum."Clear", "Color Box"=14013909}, {"Operation"=enum."Update", "Color Box"=14013909}, {"Operation"=enum."Update", "Color Box"=16777215}, {"Operation"=enum."Clear", "Color Box"=14013909}, {"Operation"=enum."Clear", "Color Box"=14013909}, {"Operation"=enum."Clear", "Color Box"=14013909}] -> [_ _ w243 _ w271]
          tunnel: w232 -> [_ _ w242 _ w270]
          tunnel: u32[] [15790320, 15790320, 15790320, 15790320, 16777215, 16777215, 15790320, 15790320, 15790320] -> [_ _ _ _ w276]
          tunnel: w230 -> [_ _ _ _ w264]
          tunnel: w227 -> [_ w237 _ _ _]
          frame "Custom", Default {
          }
          frame "Basic" {
            n121 = call <vilib>:"WPI_DashboardUpdateNames.vi"("Controls on Tab"=w237) -> ()  [unwired: 11 in]
          }
          frame "Test" {
            w249 = -2 ("Active Item:Row Number")
            n122 = Index Array(array=w243, index=w242) -> (element=w244:T23)
            n123 = Unbundle(w244) -> ("Operation"=w245:enum16{"Update", "Clear"}, "Color Box"=w246:u32)
            n124 = call <vilib>:"NT Read String.vi"("Name"="TestMode/TestName") -> ("String"=w240:string)  [unwired: 9 in, 1 out]
            n125 = call <vilib>:"NT Read and Format Entries as Tree.vi"("Operation"=w245, "Name Pattern"=w250, "Tree Refnum"=w251) -> ()  [unwired: 7 in, 2 out]
            n126 = case shown="\"\"" w240 {
              tunnel: "TestMode/TestProgress" ("Name") -> [w253 _]
              tunnel: "TestMode/TestProgressText" ("Name") -> [w252 _]
              frame Default {
                n127 = call <vilib>:"NT Read Number.vi"("Name"=w253) -> ("Numeric"=w254:dbl)  [unwired: 9 in, 1 out]
                n128 = call <vilib>:"NT Read String.vi"("Name"=w252) -> ("String"=w255:string)  [unwired: 9 in, 1 out]
                n129 = Bundle("Numeric"=w254, "String"=w255) -> (→"Progress":cluster{"Numeric":dbl, "String":string})  [unwired: 1 in]
              }
              frame "" {
                n130 = property on="Progress" class="Clust (strict)"("Visible"=FALSE) -> ()  [unwired: 2 in, 2 out]
                n131 = local write "Test Name"(u16 0) -> ()
              }
            }
            n132 = property on="Test Tree" class="Tree (strict)"("Active Item Row Number"=w249, "ActiveColNum"=w249, "CellBG"=w246, "Active Item Row Number"=-1 ("Active Item:Row Number"), "CellBG"=u32 5789784 ("Color Box")) -> ()  [unwired: 2 in, 2 out]
          }
          frame "Variables" {
            w261 = string[] ["CameraPublisher", "Usage", "DB"]  # Items to initially close
            n133 = First Call?() -> (First Call?: T/F=w262:bool)
            n134 = control-ref of="Tree"() -> (w263:refnum<vi>)
            n135 = Select(t=w261, s=w262, f=string[] []) -> (s? t:f=w259:string[])
            n136 = call <vilib>:"NT Read and Format Entries as Tree.vi"("Tags to  Close"=w259, "Tree Refnum"=w263) -> ()  [unwired: 8 in, 2 out]
          }
          frame "Commands" {
            w272 = u32 5789784 ("Color Box")
            w273 = T24 {"Row"=-1, "Column"=-2} ("Active Cell:Active Cell")
            w275 = T24 {"Row"=-2, "Column"=-2} ("Active Cell:Active Cell")
            n137 = Index Array(array=w276, index=w270) -> (element=w274:u32)
            n138 = Index Array(array=w271, index=w270) -> (element=w269:T23)
            n139 = Unbundle(w269) -> ("Operation"=w268:enum16{"Update", "Clear"})  [unwired: 1 out]
            n140 = local read "Command Selection"() -> (w267:i32)
            n141 = property on="Command Selection" class="MCListbox (strict)"("ActiveCell"=w275, "CellBG"=w274, "ActiveCell"=w273, "CellBG"=w272) -> ()  [unwired: 2 in, 2 out]
            n142 = call <vilib>:"WPI_DashboardUpdate RPC Info.vi"("Operation"=w268) -> ("update"=w266:bool, "commands"=w265:string[][])  [unwired: 9 in]
            n143 = property on="Command Selection" class="MCListbox (strict)"("ItemNames"=w265) -> ()  [unwired: 2 in, 2 out]
            n144 = property on="Command Params" class="Tbl (strict)"("Active Cell"=w275, "Cell BG Color"=w274, "Active Cell"=w273, "Cell BG Color"=w272) -> ()  [unwired: 2 in, 2 out]
            n145 = call <vilib>:"WPI_DashboardUpdate Command Params.vi"("Update"=w266, "NewVal"=w267, "Commands"=w265, "Param Tbl"=w264) -> ()  [unwired: 7 in, 1 out]
          }
        }
        n146 = call <vilib>:"Connextion Info.vi"() -> ("Connected"=→"NT Connection":bool)  [unwired: 10 in, 1 out]
      }
      event "Test Tree": Value Change {
        # "Show appropriate\ncontrols"
        n147 = event-data() -> ("CtlRef"=w281:refnum<vi>, "NewVal"=w279:string)  [unwired: 1 in]
        n148 = call <vilib>:"WPI_UtilitiesGetTreeIOName.vi"("NewVal"=w279, "TreeControl in"=w281) -> ("I/O Name"=w282:string)  [unwired: 9 in]
        n149 = case shown="\"Camera\"" w282 {
          selector: w282 -> [_ w289 _ w311 w320 _]
          tunnel: w279 -> [_ _ w308 w310 _ w327]
          tunnel: cluster{string[]}[] [{["640x480", "320x240", "160x120"]}, {["Auto", "Fixed indoor", "Fixed outdoor 1", "Fixed outdoor 2", "Fixed fluorescent 1", "Fixed fluorescent 2", "Hold current"]}, {["Auto", "Flicker-free 50 Hz", "Flicker-free 60 Hz", "Hold current"]}, {["None", "Prioritize frame rate", "Prioritize image quality"]}, {["Monochrome", "Color"]}] -> [_ _ _ _ _ w326]
          frame Default {
            w284 = FALSE ("Visible")
            w283 = FALSE ("Visible")
            n150 = property on="Motor" class="Clust (strict)"("Visible"=w283) -> ()  [unwired: 2 in, 2 out]
            n151 = property on="Test Ring" class="Ring (strict)"("Visible"=w283) -> ()  [unwired: 2 in, 2 out]
            n152 = property on="Rev/Fwd" class="Clust (strict)"("Visible"=w284) -> ()  [unwired: 2 in, 2 out]
            n153 = property on="On/Off" class="Bool (strict)"("Visible"=w284) -> ()  [unwired: 2 in, 2 out]
            n154 = property on="Test Slider" class="Slide (strict)"("Visible"=w284) -> ()  [unwired: 2 in, 2 out]
          }
          frame "Analog Out", "Motor", "PWM" {
            w290 = FALSE ("Visible")
            n155 = case shown="\"Analog Out\"" w289 {
              tunnel: [1.0 ("Value") -1.0 ("Value") 0.0 ("Value")] -> w288
              tunnel: [255.0 ("Value") 1.0 ("Value") 5.0 ("Value")] -> w287
              tunnel: [128.0 ("Value") 0.0 ("Value") 0.0 ("Value")] -> w286
              tunnel: [64.0 ("Value") 0.5 ("Value") 1.0 ("Value")] -> w285
              frame "PWM" {
              }
              frame "Motor", Default {
              }
              frame "Analog Out" {
              }
            }
            n156 = property on="Motor" class="Clust (strict)"("Visible"=TRUE) -> ()  [unwired: 2 in, 2 out]
            n157 = property on="Value" class="Slide (strict)"("Value"=w286, "Scale.Minimum"=w288, "Scale.Maximum"=w287, "Scale.Increment"=w285) -> ()  [unwired: 2 in, 2 out]
            n158 = property on="On/Off" class="Bool (strict)"("Visible"=w290) -> ()  [unwired: 2 in, 2 out]
            n159 = property on="Test Slider" class="Slide (strict)"("Visible"=w290) -> ()  [unwired: 2 in, 2 out]
            n160 = property on="Test Ring" class="Ring (strict)"("Visible"=w290) -> ()  [unwired: 2 in, 2 out]
            n161 = property on="Rev/Fwd" class="Clust (strict)"("Visible"=w290) -> ()  [unwired: 2 in, 2 out]
          }
          frame "Servo" {
            w306 = FALSE ("Visible")
            n162 = call <vilib>:"NT Read Number.vi"("Name"=w308) -> ("Numeric"=w307:dbl)  [unwired: 9 in, 1 out]
            n163 = property on="Test Slider" class="Slide (strict)"("Visible"=TRUE, "Scale.Maximum"=170.0 ("Scale.Range:Maximum")) -> ()  [unwired: 2 in, 2 out]
            n164 = local write "Test Slider"(w307) -> ()
            n165 = property on="Motor" class="Clust (strict)"("Visible"=w306) -> ()  [unwired: 2 in, 2 out]
            n166 = property on="Rev/Fwd" class="Clust (strict)"("Visible"=w306) -> ()  [unwired: 2 in, 2 out]
            n167 = property on="On/Off" class="Bool (strict)"("Visible"=w306) -> ()  [unwired: 2 in, 2 out]
            n168 = property on="Test Ring" class="Ring (strict)"("Visible"=w306) -> ()  [unwired: 2 in, 2 out]
          }
          frame "Relay", "Solenoid" {
            w309 = FALSE ("Visible")
            n169 = property on="Motor" class="Clust (strict)"("Visible"=w309) -> ()  [unwired: 2 in, 2 out]
            n170 = property on="Test Slider" class="Slide (strict)"("Visible"=w309) -> ()  [unwired: 2 in, 2 out]
            n171 = Search and Replace String(input string=w310, search string="/Value  **", replace string="/Direction") -> (result string=w316:string)  [unwired: 5 in, 3 out]
            n172 = property on="Test Ring" class="Ring (strict)"("Visible"=w309) -> ()  [unwired: 2 in, 2 out]
            n173 = call <vilib>:"NT Read String.vi"("Name"=w316) -> ("String"=w314:string)  [unwired: 9 in, 1 out]
            n174 = Equal?(x="Both directions", y=w314) -> (x = y?=w312:bool)
            n175 = Not(x=w312) -> (.not. x?=w313:bool)
            n176 = property on="Rev/Fwd" class="Clust (strict)"("Visible"=w312) -> ()  [unwired: 2 in, 2 out]
            n177 = property on="On/Off" class="Bool (strict)"("Visible"=w313, "Caption.Text"=w311) -> ()  [unwired: 2 in, 2 out]
          }
          frame "Compressor", "Digital Out" {
            w319 = FALSE ("Visible")
            # "Get direction and finish"
            n178 = property on="Motor" class="Clust (strict)"("Visible"=w319) -> ()  [unwired: 2 in, 2 out]
            n179 = property on="Test Slider" class="Slide (strict)"("Visible"=w319) -> ()  [unwired: 2 in, 2 out]
            n180 = property on="Test Ring" class="Ring (strict)"("Visible"=w319) -> ()  [unwired: 2 in, 2 out]
            n181 = property on="On/Off" class="Bool (strict)"("Visible"=TRUE, "Caption.Text"=w320) -> ()  [unwired: 2 in, 2 out]
            n182 = property on="Rev/Fwd" class="Clust (strict)"("Visible"=FALSE) -> ()  [unwired: 2 in, 2 out]
          }
          frame "Camera" {
            n183 = call <vilib>:"Get Last Path Segment.vi"("String in"=w327) -> ("String out"=w328:string)  [unwired: 10 in]
            n184 = property on="On/Off" class="Bool (strict)"("Visible"=FALSE) -> ()  [unwired: 2 in, 2 out]
            n185 = property on="Motor" class="Clust (strict)"("Visible"=FALSE) -> ()  [unwired: 2 in, 2 out]
            n186 = property on="Rev/Fwd" class="Clust (strict)"("Visible"=FALSE) -> ()  [unwired: 2 in, 2 out]
            n187 = case shown="\"White Balance  **\"" w328 {
              tunnel: w327 -> [w334 w343 w352 w361 w370 _ w376]
              tunnel: w326 -> [w332 w340 w349 w358 w367 _ _]
              frame "Size  **" {
                n188 = Index Array(array=w332) -> (element=w331:cluster{string[]})  [unwired: 1 in]
                n189 = call <vilib>:"NT Read String.vi"("Name"=w334) -> ("String"=w333:string)  [unwired: 9 in, 1 out]
                n190 = Unbundle(w331) -> (w329:string[])
                n191 = Match First String(2:w329, 3:w333) -> (0:w330:i32)  [unwired: 1 out]
                n192 = property on="Test Ring" class="Ring (strict)"("Value"=w330, "Strings []"=w329) -> ()  [unwired: 2 in, 2 out]
                n193 = property on="Test Ring" class="Ring (strict)"("Visible"=TRUE) -> ()  [unwired: 2 in, 2 out]
                n194 = property on="Test Slider" class="Slide (strict)"("Visible"=FALSE) -> ()  [unwired: 2 in, 2 out]
              }
              frame "White Balance  **" {
                n195 = Index Array(array=w340, index=1) -> (element=w341:cluster{string[]})
                n196 = call <vilib>:"NT Read String.vi"("Name"=w343) -> ("String"=w342:string)  [unwired: 9 in, 1 out]
                n197 = Unbundle(w341) -> (w338:string[])
                n198 = Match First String(2:w338, 3:w342) -> (0:w337:i32)  [unwired: 1 out]
                n199 = property on="Test Ring" class="Ring (strict)"("Value"=w337, "Strings []"=w338) -> ()  [unwired: 2 in, 2 out]
                n200 = property on="Test Ring" class="Ring (strict)"("Visible"=TRUE) -> ()  [unwired: 2 in, 2 out]
                n201 = property on="Test Slider" class="Slide (strict)"("Visible"=FALSE) -> ()  [unwired: 2 in, 2 out]
              }
              frame "Exposure  **" {
                n202 = Index Array(array=w349, index=2) -> (element=w350:cluster{string[]})
                n203 = call <vilib>:"NT Read String.vi"("Name"=w352) -> ("String"=w351:string)  [unwired: 9 in, 1 out]
                n204 = Unbundle(w350) -> (w346:string[])
                n205 = Match First String(2:w346, 3:w351) -> (0:w347:i32)  [unwired: 1 out]
                n206 = property on="Test Ring" class="Ring (strict)"("Value"=w347, "Strings []"=w346) -> ()  [unwired: 2 in, 2 out]
                n207 = property on="Test Ring" class="Ring (strict)"("Visible"=TRUE) -> ()  [unwired: 2 in, 2 out]
                n208 = property on="Test Slider" class="Slide (strict)"("Visible"=FALSE) -> ()  [unwired: 2 in, 2 out]
              }
              frame "Exposure Priority  **" {
                n209 = Index Array(array=w358, index=3) -> (element=w359:cluster{string[]})
                n210 = call <vilib>:"NT Read String.vi"("Name"=w361) -> ("String"=w360:string)  [unwired: 9 in, 1 out]
                n211 = Unbundle(w359) -> (w355:string[])
                n212 = Match First String(2:w355, 3:w360) -> (0:w356:i32)  [unwired: 1 out]
                n213 = property on="Test Ring" class="Ring (strict)"("Value"=w356, "Strings []"=w355) -> ()  [unwired: 2 in, 2 out]
                n214 = property on="Test Ring" class="Ring (strict)"("Visible"=TRUE) -> ()  [unwired: 2 in, 2 out]
                n215 = property on="Test Slider" class="Slide (strict)"("Visible"=FALSE) -> ()  [unwired: 2 in, 2 out]
              }
              frame "Color Enable  **" {
                n216 = Index Array(array=w367, index=4) -> (element=w368:cluster{string[]})
                n217 = call <vilib>:"NT Read String.vi"("Name"=w370) -> ("String"=w369:string)  [unwired: 9 in, 1 out]
                n218 = Unbundle(w368) -> (w364:string[])
                n219 = Match First String(2:w364, 3:w369) -> (0:w365:i32)  [unwired: 1 out]
                n220 = property on="Test Ring" class="Ring (strict)"("Value"=w365, "Strings []"=w364) -> ()  [unwired: 2 in, 2 out]
                n221 = property on="Test Ring" class="Ring (strict)"("Visible"=TRUE) -> ()  [unwired: 2 in, 2 out]
                n222 = property on="Test Slider" class="Slide (strict)"("Visible"=FALSE) -> ()  [unwired: 2 in, 2 out]
              }
              frame Default {
                n223 = property on="Test Ring" class="Ring (strict)"("Visible"=FALSE) -> ()  [unwired: 2 in, 2 out]
                n224 = property on="Test Slider" class="Slide (strict)"("Visible"=FALSE) -> ()  [unwired: 2 in, 2 out]
              }
              frame "Brightness  **", "Color Level  **", "Compression  **", "FPS  **", "Sharpness  **" {
                n225 = call <vilib>:"NT Read Number.vi"("Name"=w376) -> ("Numeric"=w375:dbl)  [unwired: 9 in, 1 out]
                n226 = local write "Test Slider"(w375) -> ()
                n227 = property on="Test Slider" class="Slide (strict)"("Visible"=TRUE, "Scale.Maximum"=100.0 ("Scale.Range:Maximum")) -> ()  [unwired: 2 in, 2 out]
                n228 = property on="Test Ring" class="Ring (strict)"("Visible"=FALSE) -> ()  [unwired: 2 in, 2 out]
              }
            }
          }
        }
        n229 = property on="Progress" class="Clust (strict)"("Visible"=FALSE) -> ()  [unwired: 2 in, 2 out]
      }
      event "Test Name": Mouse Enter {
        # "Populate the ring with the list of tests"
        n230 = event-data() -> ()  [unwired: 1 in, 1 out]
        n231 = call <vilib>:"NT Read String Array.vi"("Name"="TestMode/TestList") -> ("String Array"=w384:string[])  [unwired: 9 in, 1 out]
        n232 = Build Array (concatenate)("Select the test to run...", w384) -> (w383:string[])
        n233 = property on="Test Name" class="Ring (strict)"("Strings []"=w383) -> ()  [unwired: 2 in, 2 out]
      }
      event "Test Name": Value Change {
        w386 = FALSE ("Visible")
        # "Tell the robot the test name to run"
        n234 = event-data() -> ("NewVal"=w390:u16)  [unwired: 1 in]
        n235 = property on="Test Name" class="Ring (strict)"() -> ("Strings []"=w391:string[])  [unwired: 2 in, 2 out]
        n236 = local write "Progress"(T6 {"Test Progress"=0, "Test Progress Text"=""} ("Progress")) -> ()
        n237 = Index Array(array=w391, index=w390) -> (element=w389:string)
        n238 = call <vilib>:"NT Write String.vi"("String"=w389, "Name"="TestMode/TestName") -> ()  [unwired: 9 in, 1 out]
        n239 = property on="Progress" class="Clust (strict)"("Visible"=TRUE) -> ()  [unwired: 2 in, 2 out]
        n240 = property on="Motor" class="Clust (strict)"("Visible"=w386) -> ()  [unwired: 2 in, 2 out]
        n241 = property on="Test Slider" class="Slide (strict)"("Visible"=w386) -> ()  [unwired: 2 in, 2 out]
        n242 = property on="On/Off" class="Bool (strict)"("Visible"=w386) -> ()  [unwired: 2 in, 2 out]
        n243 = property on="Rev/Fwd" class="Clust (strict)"("Visible"=w386) -> ()  [unwired: 2 in, 2 out]
        n244 = property on="Test Ring" class="Ring (strict)"("Visible"=w386) -> ()  [unwired: 2 in, 2 out]
      }
      event "Select Auto": Mouse Enter {
        # "Populate the combo box with the list of autonomous options"
        n245 = event-data() -> ()  [unwired: 1 in, 1 out]
        n246 = call <vilib>:"NT Read String Array.vi"("Name"="Auto List2") -> ("String Array"=w393:string[])  [unwired: 9 in, 1 out]
        n247 = property on="Select Auto" class="CmbBox"("Strings[]"=w393) -> ()  [unwired: 2 in, 2 out]
      }
      event "Select Auto": Value Change {
        # "User modified the Auto Selection. Write to NT variable so robot knows."
        n248 = event-data() -> ("NewVal"=w396:string)  [unwired: 1 in]
        n249 = call <vilib>:"NT Write String.vi"("String"=w396, "Name"="Auto Selector") -> ()  [unwired: 9 in, 1 out]
      }
      event "Command Selection": Value Change {
        # "Get the params and show in table"
        n250 = event-data() -> ("NewVal"=w402:i32)  [unwired: 1 in]
        n251 = property on="Command Selection" class="MCListbox (strict)"() -> ("ItemNames"=w400:string[][])  [unwired: 2 in, 2 out]
        n252 = call <vilib>:"WPI_DashboardUpdate Command Params.vi"("NewVal"=w402, "Commands"=w400, "Param Tbl"=w401) -> ()  [unwired: 8 in, 1 out]
      }
      event "Execute Command": Value Change {
        # "Started one, Unique ID holds\nresponse"
        n253 = event-data() -> ()  [unwired: 1 in, 1 out]
        n254 = property on="Command Selection" class="MCListbox (strict)"() -> ("ItemNames"=w413:string[][])  [unwired: 2 in, 2 out]
        n255 = Index Array(array=w413, index (row)="Command Selection", index (col)=0) -> (element=w411:string)
        n256 = call <vilib>:"Invoke Commands.vi"("Command Params"="Command Params", "Function Name"=w411) -> ("Params"=w407:u8, "Started"=w406:bool)  [unwired: 7 in, 1 out]
        n257 = Array Subset(array="Command Params", length (row)=w407) -> (w408:string[][])  [unwired: 3 in]
        n258 = Select(t="Executing" ("Cmd Status"), s=w406, f="" ("Cmd Status")) -> (s? t:f=→"Cmd Status":string)
      }
      event "Command Selection": Double Click {
        n259 = event-data() -> ("Row"=w421:i32)  [unwired: 1 in]
        n260 = property on="Command Selection" class="MCListbox (strict)"() -> ("ItemNames"=w424:string[][])  [unwired: 2 in, 2 out]
        n261 = local read "Command Params"() -> (w420:string[][])
        n262 = Index Array(array=w424, index (row)=w421, index (col)=0) -> (element=w422:string)
        n263 = call <vilib>:"Invoke Commands.vi"("Command Params"=w420, "Function Name"=w422) -> ("Params"=w419:u8, "Started"=w414:bool)  [unwired: 7 in, 1 out]
        n264 = Array Subset(array=w420, length (row)=w419) -> (w418:string[][])  [unwired: 3 in]
        n265 = Select(t="Executing" ("Cmd Status"), s=w414, f="" ("Cmd Status")) -> (s? t:f=w415:string)
        n266 = local write "Cmd Status"(w415) -> ()
      }
      event "CheckList": Double Click {
        # "Shift clears all"
        # "Update symbols on the listbox"
        n267 = event-data() -> ("PlatMods.Shift"=w426:bool, "Row"=w428:i32)  [unwired: 1 in]
        n268 = case shown="True" w426 {
          tunnel: w428 -> [w432 _]
          tunnel: 1 -> [w431 _]
          frame False {
            n269 = property on="CheckList" class="LstBox (strict)"() -> ("Item Symbols"=w430:i32[])  [unwired: 2 in, 2 out]
            n270 = Replace Array Subset(array=w430, new element=w431, index=w432) -> (w429:i32[])
            n271 = property on="CheckList" class="LstBox (strict)"("Item Symbols"=w429) -> ()  [unwired: 2 in, 2 out]
          }
          frame True {
            w433 = 0 ("Top Row")
            n272 = property on="CheckList" class="LstBox (strict)"() -> ("Number of Rows"=w435:u32)  [unwired: 2 in, 2 out]
            n273 = Initialize Array(0, w435) -> (w434:i32[])
            n274 = property on="CheckList" class="LstBox (strict)"("Top Row"=w433, "Value"=w433, "Item Symbols"=w434) -> ()  [unwired: 2 in, 2 out]
          }
        }
      }
      event "CheckList": Key Down {
        # "Update symbols on the listbox\nLeft and right keys check and uncheck"
        n275 = event-data() -> ("VKey"=w439:T21)  [unwired: 1 in]
        n276 = case shown="\"Left\", \"Right\"" w439 {
          selector: w439 -> [w444 _]
          tunnel: eventvkey."Left" ("VKey") -> [w442 _]
          frame "Left", "Right" {
            n277 = Equal?(x=w442, y=w444) -> (x = y?=w443:bool)
            n278 = Select(t=0, s=w443, f=1) -> (s? t:f=w445:i32)
            n279 = property on="CheckList" class="LstBox (strict)"() -> ("Item Symbols"=w448:i32[])  [unwired: 2 in, 2 out]
            n280 = Replace Array Subset(array=w448, new element=w445, index="CheckList") -> (w447:i32[])
            n281 = property on="CheckList" class="LstBox (strict)"("Item Symbols"=w447) -> ()  [unwired: 2 in, 2 out]
          }
          frame Default {
          }
        }
      }
      event "Motor.Enable": Value Change {
        # "When the test mode otor enable helper is set, update that\ntree row item's value"
        n282 = event-data() -> ("NewVal"=w454:bool)  [unwired: 1 in]
        n283 = Unbundle("Motor") -> ("Value"=w453:dbl)  [unwired: 1 out]
        n284 = Select(t=w453, s=w454, f=0.0) -> (s? t:f=w451:dbl)
        n285 = call <vilib>:"NT Write Number.vi"("Numeric"=w451, "Name"=w450) -> ()  [unwired: 9 in, 1 out]
      }
      event "Test Slider": Value Change {
        # "When the test mode slider helper is set, update that\ntree row item's value"
        n286 = event-data() -> ("NewVal"=w457:dbl)  [unwired: 1 in]
        n287 = call <vilib>:"NT Write Number.vi"("Numeric"=w457, "Name"=w458) -> ()  [unwired: 9 in, 1 out]
      }
      event "On/Off": Value Change {
        # "When the test mode on/off helper value is set, update that\ntree row item's value"
        n288 = event-data() -> ("NewVal"=w462:bool)  [unwired: 1 in]
        n289 = Boolean To (0,1)(Boolean=w462) -> (0, 1=w461:i16)
        n290 = call <vilib>:"NT Write Number.vi"("Numeric"=w461, "Name"=w460) -> ()  [unwired: 9 in, 1 out]
      }
      event "Rev/Fwd": Value Change {
        # "When the test mode helper value for relays is set, update that\ntree row item's value"
        n291 = event-data() -> ("NewVal.Forward"=w470:bool, "NewVal.Reverse"=w469:bool)  [unwired: 1 in]
        n292 = Boolean To (0,1)(Boolean=w470) -> (0, 1=w466:i16)
        n293 = Boolean To (0,1)(Boolean=w469) -> (0, 1=w468:i16)
        n294 = Negate(x=w468) -> (-x=w467:i16)
        n295 = Add(x=w466, y=w467) -> (x+y=w465:i16)
        n296 = call <vilib>:"NT Write Number.vi"("Numeric"=w465, "Name"=w464) -> ()  [unwired: 9 in, 1 out]
      }
      event "Test Ring": Value Change {
        # "When a test mode helper value is selected from the ring,\nset the tree item's variable to the string value"
        n297 = event-data() -> ("NewVal"=w474:u16)  [unwired: 1 in]
        n298 = property on="Test Ring" class="Ring (strict)"() -> ("Strings []"=w475:string[])  [unwired: 2 in, 2 out]
        n299 = Index Array(array=w475, index=w474) -> (element=w473:string)
        n300 = call <vilib>:"NT Write String.vi"("String"=w473, "Name"=w472) -> ()  [unwired: 9 in, 1 out]
      }
      event "Rec Mode": Value Change {
        # "Update globals for recording mode and path to read log from.\nClear when logging and let NetworkTables set path for vision to\nuse."
        n301 = event-data() -> ("NewVal"=w486:enum32{"Stop", "Record", "Playback"})  [unwired: 1 in]
        n302 = global write "WPI_DashboardLogging Global.vi" "Logging Filename"(path "") -> ()
        n303 = global write "WPI_DashboardLogging Global.vi" "Recording"(w486) -> ()
        n304 = case shown="\"Playback\"" w486 {
          tunnel: w485 -> [_ w488 w497]
          tunnel: [_ _ w496] -> w483
          tunnel: [_ _ w495] -> _
          tunnel: w481 -> [_ _ w493]
          tunnel: cluster{i32, i32} {-250, 170} -> [_ _ w492]
          tunnel: [_ _ T22 {"Image Size"=TRUE, "Image Type"=TRUE, "Pixel Value"=TRUE, "ROI Information"=TRUE, "Zoom Factor"=FALSE} ("Image Information Shown:All Elements")] -> w476
          tunnel: [_ _ TRUE ("Zoom Factor")] -> w477
          tunnel: w479 -> [_ _ w489]
          frame Default {
          }
          frame "Stop", "Record" {
            # "Place Window too"
            n305 = invoke class="VI" method="FP.Close"(reference=w488) -> (reference out=w487:refnum<vi>)  [unwired: 2 in, 2 out]
            n306 = invoke class="VI" method="Abort VI"(reference=w487) -> ()  [unwired: 2 in, 3 out]
          }
          frame "Playback" {
            n307 = call "Open Playback Panel.vi"("Offset"=w492, "DB VI Ref"=w493, "Playback in"=w497) -> ("Playback out"=w494:refnum<vi>)  [unwired: 8 in]
            n308 = register-events(w494, w489) -> (reference out=w496:refnum<event-registration>, error out=w495:errorcluster)  [unwired: 2 in]
          }
        }
        n309 = property on="Camera Image Right" class="ImageControl"("Image Information Shown"=w476, "Image Information Visible"=w477) -> ()  [unwired: 2 in, 2 out]
        n310 = property on="Camera Image" class="ImageControl"("Image Information Shown"=w476, "Image Information Visible"=w477) -> ()  [unwired: 2 in, 2 out]
        n311 = call <vilib>:"WPI_DashboardNT Log FieldName Cache.vi"("Operation"=enum16{"Lookup/Add", "Index", "Clear"}."Clear") -> ()  [unwired: 8 in, 3 out]
      }
      event Panel Close {
        w499 = enum32{"Stop", "Record", "Playback"}."Stop" ("Rec Mode")
        # "Playback window has been closed, abort"
        n312 = event-data() -> ()  [unwired: 1 in, 4 out]
        n313 = local write "Rec Mode"(w499) -> ()
        n314 = global write "WPI_DashboardLogging Global.vi" "Recording"(w499) -> ()
      }
      event Panel Close {
        # "Abort playback window and ourself"
        n315 = event-data() -> ()  [unwired: 1 in, 4 out]
        n316 = invoke class="VI" method="FP.Close"(reference=w503) -> (reference out=w502:refnum<vi>)  [unwired: 2 in, 2 out]
        n317 = invoke class="VI" method="Abort VI"(reference=w502) -> (error out=w501:errorcluster)  [unwired: 2 in, 2 out]
        n318 = invoke class="VI" method="Abort VI"(error in=w501) -> ()  [unwired: 2 in, 3 out]
      }
      event User Event {
        n319 = event-data() -> ("IDs"=w510:cluster{"RPC field ID":u16, "Unique ID":u16}, "String"=w509:string)  [unwired: 1 in]
        n320 = Bundle("IDs"=w510, "String"=w509) -> (w508:T9)  [unwired: 1 in]
        n321 = call <vilib>:"Retrieve RPC Response.vi"("RPC Response"=w508) -> ("Output"=w506:string[][])  [unwired: 10 in]
        n322 = Build Array (concatenate)(w504, w506) -> (w505:string[][])
        n323 = local write "Command Params"(w505) -> ()
        n324 = local write "Cmd Status"("" ("Cmd Status")) -> ()
      }
      event "Tree": Double Click {
        n325 = event-data() -> ("PlatMods"=w516:T25, "Tag"=w513:string)  [unwired: 1 in]
        n326 = Unbundle(w516) -> ("Shift"=w515:bool)  [unwired: 4 out]
        n327 = String Subset(string=w513, length (rest)=1 ("length (rest)")) -> (substring=w512:string)  [unwired: 1 in]
        n328 = Not(x=w515) -> (.not. x?=w514:bool)
        n329 = case shown="\"/\"" w512 {
          tunnel: w513 -> [_ w519]
          tunnel: w514 -> [_ w518]
          frame Default {
          }
          frame "/" {
            n330 = call <vilib>:"NT Update Persistence.vi"("Persistence"=w518, "Name"=w519) -> ()  [unwired: 9 in, 1 out]
          }
        }
      }
    }
  }
  n331 = while {
    tunnel: w65 -> [w521]
    i -> [w524]
    stop <- FALSE stop-if-true
    n332 = Wait (ms)(milliseconds to wait=u32 100) -> ()  [unwired: 1 out]
    n333 = case shown="\"Playback\"" "Rec Mode" {
      tunnel: w524 -> [_ _ w539]
      tunnel: [u32 2829099 ("Base Color") u32 11141120 ("Target Color") w528] -> w520
      frame "Stop", Default {
        # "Reset the color, extra updates don't cost much"
      }
      frame "Record" {
      }
      frame "Playback" {
        # "Playback"
        n334 = Quotient & Remainder(x=w539, y=u32 50 ("milliseconds to wait")) -> (x-y*floor(x/y)=w535:u32)  [unwired: 1 out]
        n335 = Divide(x=w535, y=u32 50 ("milliseconds to wait")) -> (x/y=w532:dbl)
        n336 = Multiply(x=6.283185307179586, y=w532) -> (x*y=w537:dbl)
        n337 = Sine(x=w537) -> (sin(x)=w536:dbl)
        n338 = Absolute Value(x=w536) -> (abs(x)=w529:dbl)
        n339 = call "Interpolate RGB Color.vi"("Proportion"=w529, "Target Color"=u32 30976, "Base Color"=u32 2829099) -> ("Result Color"=w528:u32)  [unwired: 8 in]
      }
    }
    n340 = property class="Pane"(reference=w521, "PaneColor"=w520) -> ()  [unwired: 1 in, 2 out]
  }
  n341 = local write "Dashboard Tab"(T2."Drive" ("Dashboard Tab")) -> ()
  n342 = property on="On/Off" class="Bool (strict)"("Visible"=w36) -> ()  [unwired: 2 in, 2 out]
  n343 = property on="Motor" class="Clust (strict)"("Visible"=w36) -> ()  [unwired: 2 in, 2 out]
  n344 = property on="Progress" class="Clust (strict)"("Visible"=w36) -> ()  [unwired: 2 in, 2 out]
  n345 = property on="Test Ring" class="Ring (strict)"("Visible"=w36) -> ()  [unwired: 2 in, 2 out]
  n346 = property on="Rev/Fwd" class="Clust (strict)"("Visible"=w36) -> ()  [unwired: 2 in, 2 out]
  n347 = while {
    tunnel: u16 1741 ("timeout ms (25000)") -> [w541]
    stop <- FALSE stop-if-true
    n348 = TCP Create Listener(10:w541) -> (0:w540:errorcluster, 3:w542:refnum<k5>)  [unwired: 4 in, 1 out]
    n349 = case shown="No Error" w540 {
      selector: w540 -> [w544 _]
      tunnel: w542 -> [w545 _]
      frame No Error {
        n350 = while {
          tunnel: w545 -> [w548]
          tunnel: w544 -> [w547]
          stop <- FALSE stop-if-true
          n351 = TCP Wait On Listener(8:w547, 11:w548) -> (0:w549:errorcluster, 4:w550:refnum<k5>)  [unwired: 2 in, 3 out]
          n352 = local write "TCP"(w550) -> ()
          n353 = case shown="No Error" w549 {
            frame No Error {
            }
            frame Error {
              n354 = Wait (ms)(milliseconds to wait=u32 1000) -> ()  [unwired: 1 out]
            }
          }
        }
      }
      frame Error {
        n355 = Wait (ms)(milliseconds to wait=u32 1000) -> ()  [unwired: 1 out]
      }
    }
  }
  n356 = local write "Command Selection"(u16 0 ("milliseconds to wait")) -> ()
  n357 = local write "Command Params"(string[][] [] ("Command Params")) -> ()
  n358 = global write "WPI_DashboardLogging Global.vi" "Recording"(w59) -> ()
  n359 = local write "Rec Mode"(w59) -> ()
  n360 = call <vilib>:"NT Write String.vi"("String"="Select Auto", "Name"="Auto Selector") -> ()  [unwired: 9 in, 1 out]
